vi "Convert Bertec CSV into dynamic data type  iso.vi"(0 "selected path":path, 1 "Input Datafile Separator":enum32{"CSV", "TSV"}(radio)) -> (2 "Dynamic Data Type":dynamicdata(waveform))   [LabVIEW 2016]
uses:
  <vilib>/Utility/file.llb/Read Delimited Spreadsheet (DBL).vi
  <vilib>/Utility/file.llb/Read Delimited Spreadsheet (string).vi
panel:
  out "Dynamic Data Type 2":dynamicdata(graph)
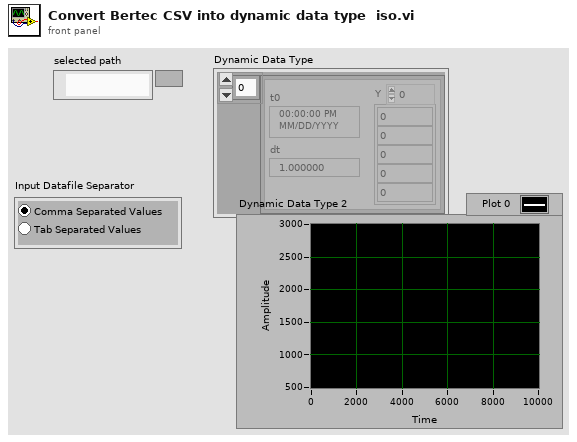
[diagram p1: front panel]
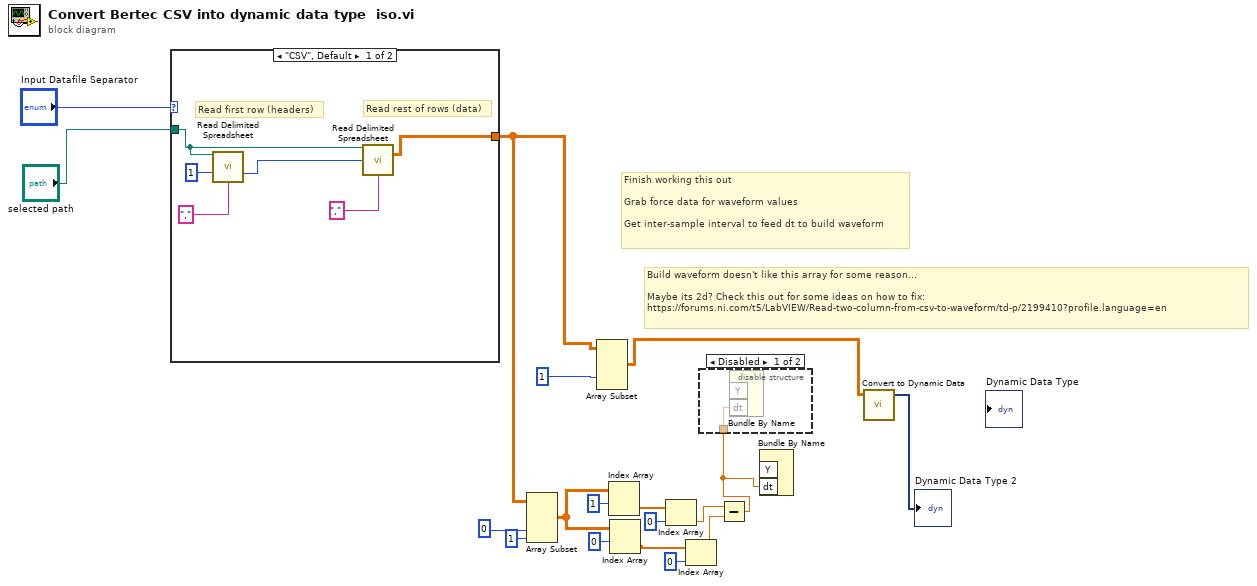
[diagram p0: block diagram]
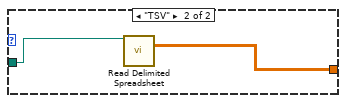
[diagram p3: hidden frame]
diagram:
  # "Build waveform doesn't like this array for some reason...\n\nMaybe its 2d? Check this out for some ideas on how to fix: \nhttps://forums.ni.com/t5/LabVIEW/Read-two-column-from-csv-to-waveform/td-p/2199410?profile.language=en"
  # "Finish working this out \n\nGrab force data for waveform values\n\nGet inter-sample interval to feed dt to build waveform"
  n1 = case shown="\"CSV\", Default" "Input Datafile Separator" {
    tunnel: "selected path" -> [w22 w26]
    tunnel: [w23 w25] -> w13
    frame "CSV", Default {
      # "Read rest of rows (data)"
      # "Read first row (headers)"
      n2 = call-poly <vilib>:"Read Delimited Spreadsheet.vi"("file path (dialog if empty)"=w22, "number of rows (all:-1)"=1, "delimiter (\\t)"="," ("delimiter (\\t)")) -> ("mark after read (chars.)"=w20:i32)  [unwired: 7 in, 5 out]
      n3 = call-poly <vilib>:"Read Delimited Spreadsheet.vi"("file path (dialog if empty)"=w22, "start of read offset (chars.:0)"=w20, "delimiter (\\t)"="," ("delimiter")) -> ("all rows"=w23:dbl[][])  [unwired: 7 in, 5 out]
    }
    frame "TSV" {
      n4 = call-poly <vilib>:"Read Delimited Spreadsheet.vi"("file path (dialog if empty)"=w26) -> ("all rows"=w25:dbl[][])  [unwired: 9 in, 5 out]
    }
  }
  n5 = Array Subset(array=w13, index (col)=0 ("index (row)"), length (col)=1 ("length")) -> (w12:dbl[][])  [unwired: 2 in]
  n6 = Array Subset(array=w13, index (col)=1 ("index (row)")) -> (w9:dbl[][])  [unwired: 3 in]
  n7 = Index Array(array=w12, index (row)=1 ("index")) -> (element=w7:dbl[])  [unwired: 1 in]
  n8 = Index Array(array=w12, index (row)=0 ("index")) -> (element=w3:dbl[])  [unwired: 1 in]
  n9 = Index Array(array=w7, index=0) -> (element=w5:dbl)
  n10 = Index Array(array=w3, index=0) -> (element=w2:dbl)
  n11 = Subtract(x=w5, y=w2) -> (x-y=w1:dbl)
  n12 = disable-structure shown="Disabled" {
    disable-tunnel: w1 -> [w27 _]
    frame Disabled {
      n13 = Bundle By Name("dt"=w27) -> ()  [unwired: 2 in, 1 out]
    }
    frame Enabled {
    }
  }
  n14 = Bundle By Name("dt"=w1) -> ()  [unwired: 2 in, 1 out]
  n15 = call "Convert to Dynamic Data"("2D Array"=w9) -> ("Dynamic Data Type"=→"Dynamic Data Type 2":dynamicdata)  [unwired: 3 in]
